vi "q1 sum odd numbers while loop.vi"() -> ()   [LabVIEW 2025]
panel:
  out "sum odd \nwhile":dbl
  in  "n":dbl
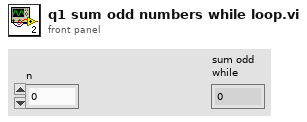
[diagram p1: front panel]
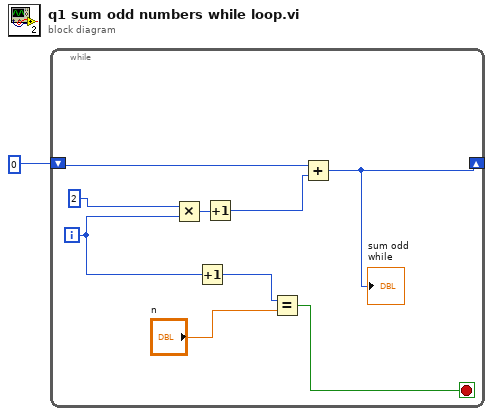
[diagram p0: block diagram]
diagram:
  n1 = while {
    shift-right: [w7] -> _
    shift-left: 0 -> [w10]
    i -> [w4]
    stop <- w6 stop-if-true
    n2 = Multiply(x=2, y=w4) -> (x*y=w3:i32)
    n3 = Increment(x=w4) -> (x+1=w8:i32)
    n4 = Increment(x=w3) -> (x+1=w2:i32)
    n5 = Equal?(x=w8, y="n") -> (x = y?=w6:bool)
    n6 = Add(x=w10, y=w2) -> (x+y=w7:i32)
    "sum odd \nwhile" <- w7
  }
